vi "Write Asserted.vi"(10 "Asserted":bool, 11 "Properties.Assert in":refnum<class "Properties.Assert.lvclass">) -> (3 "Properties.Assert out":refnum<class "Properties.Assert.lvclass">)   [LabVIEW 2013, in "Caraya.lvlib" / "Properties.Assert.lvclass"]
uses:
  Properties.Assert.lvclass
  Properties.Assert.lvclass/Properties.Assert.ctl
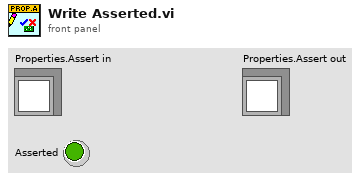
[diagram p1: front panel]
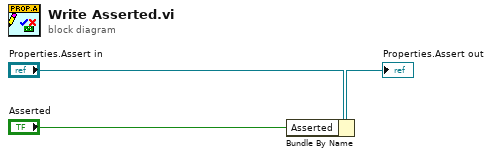
[diagram p0: block diagram]
diagram:
  n1 = Bundle By Name(cluster="Properties.Assert in", "Asserted"="Asserted") -> (→"Properties.Assert out":refnum<class "Properties.Assert.lvclass">)
